vi "Results to Text.vi"(1 "Result Array":T1[](array[typedef]) {"Test Paramaters"."Measurement res." format="%.0f MHz"; "Test Paramaters"."Blocking Signal" format="%#_gdBm"; "Test Paramaters"."Interference sig. freq." format="%.0f MHz"; "Test Paramaters"."Wanted Signal" format="%#_gdBm"; "Test Frequency" format="%.0f MHz"}) -> (0 "String":string)   [LabVIEW 2013]
doc: "This VI takes some results and converts them into text, ready for saving."
uses:
  Test Results Cluster.ctl
  Test Parameters.ctl
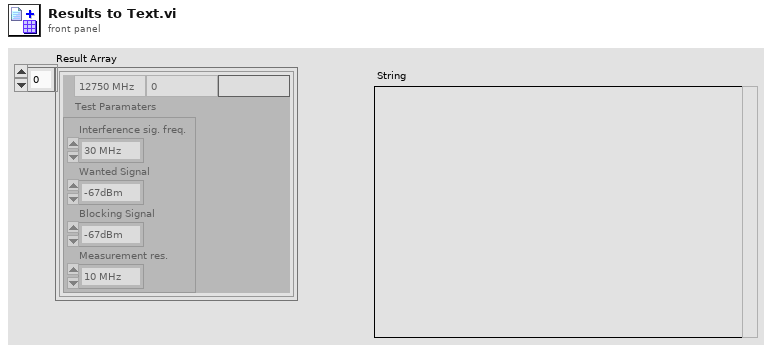
[diagram p1: front panel]
types:
  T1 = typedef "Test Results Cluster.ctl" = cluster{"Test Frequency":u32, "Received Packets":u32, "Results":string, "Test Paramaters":T2}
  T2 = typedef "Test Parameters.ctl" = cluster{"Interference sig. freq.":u32, "Wanted Signal":dbl, "Blocking Signal":dbl, "Measurement res.":u32}
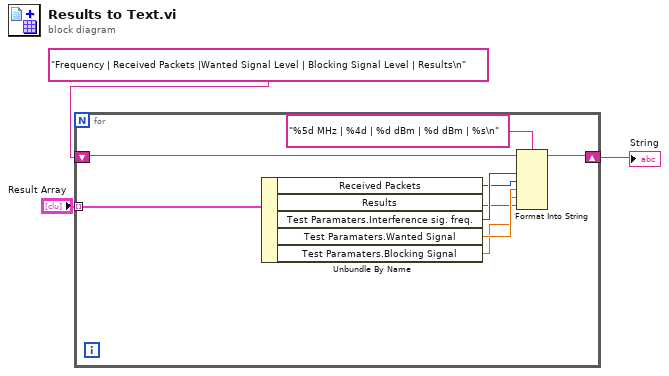
[diagram p0: block diagram]
diagram:
  n1 = for {
    tunnel: "Result Array" -> [w12] mode=indexing
    shift-right: [w10] -> w1
    shift-left: "Frequency | Received Packets |Wanted Signal Level | Blocking Signal Level | Results\n" ("format string") -> [w11]
    n2 = Unbundle By Name(w12) -> ("Received Packets"=w7:u32, "Results"=w4:string, "Test Paramaters.Interference sig. freq."=w8:u32, "Test Paramaters.Wanted Signal"=w6:dbl, "Test Paramaters.Blocking Signal"=w5:dbl)
    n3 = Format Into String(format string="%5d MHz | %4d | %d dBm | %d dBm | %s\n", initial string=w11, w8, w7, w6, w5, w4) -> (resulting string=w10:string)  [unwired: 1 in, 1 out]
  }
  "String" <- w1
